vi "Event Handler.vi"(0 "uService Template in":refnum<class "Kasli Server.lvclass">, 5 "Event type":T1=enum."Message", 7 "Item Name":string, 9 "Data":variant, 11 "error in (no error)":errorcluster) -> (4 "uService Template out":refnum<class "Kasli Server.lvclass">, 15 "error out":errorcluster)   [LabVIEW 2020, in "Kasli Server.lvlib" / "Kasli Server.lvclass"]
uses:
  Kasli Server.lvclass
  C:/Users/marco/Documents/GitHub_Lab/TALOS/talos/Father of all uServices/Father of all uServices/Father of all uServices.lvclass
  Father of all uServices/Father of all uServices/Event Handler Items.ctl
  Ancestor/Ancestor/Ancestor.lvclass/Ancestor.ctl
  Kasli Server Consumer Case Selector.ctl
  Father of all uServices/Father of all uServices Messages/Consumer Msg/Consumer Msg.lvclass/Consumer Msg.ctl
  FGV/Error Memory/Get Error Description.vi
  Support VIs/Get PC name.vi
  Ancestor/Ancestor/Read ID.vi
  Support VIs/Get Class Name.vi
  <vilib>/Utility/error.llb/Clear Errors.vi
  Father of all uServices/Father of all uServices Messages/Consumer Msg/Send Consumer.vi
  Support VIs/Substitute Error.vi
  FGV/Error Memory/Error Memory Core.vi
  <vilib>/AdvancedString/Delimited String to 1D String Array.vi
  Support VIs/Circus Root Path.vi
  FGV/Error Memory/Error Crt Lvl checker.vi
  FGV/Error Memory/Error Memory Core.vi/40c8088d-b597-4017-91af-faa98e00292e.vi
  FGV/Error Memory/Error Memory Core.vi/d4a3ab98-063c-4e44-b43d-fbdcfe6c2be2.vi
  Father of all uServices/Father of all uServices/Father of all uServices.lvclass
  C:/Users/marco/Documents/GitHub_Lab/TALOS/builds/Actor Framework PPL/Actor Framework.lvlibp/1abvi3w/vi.lib/ActorFramework/Actor/Actor.lvclass
  Support VIs/Global Memory.vi
  <vilib>/Utility/LVClass/Get LV Class Name.vi
  Support VIs/Is in Packed Library.vi
  Support VIs/TALOS Root path.vi
  Support VIs/Read CSV worksheet.vi
  Support VIs/Global Constants.vi
  <vilib>/Utility/error.llb/General Error Handler.vi
  Father of all uServices/Father of all uServices/Children Methods/Get GUI Item Value - String.vi
  builds/Actor Framework PPL/Actor Framework.lvlibp/1abvi3w/vi.lib/ActorFramework/Actor/Read Self Enqueuer.vi
  <userlib>/_OpenG.lib/lvdata/lvdata.llb/Get Strings from Enum__ogtk.vi
  builds/Actor Framework PPL/Actor Framework.lvlibp/1abvi3w/vi.lib/ActorFramework/Message Enqueuer/Enqueue.vi
  Support VIs/Error Log.vi
  Ancestor/Ancestor/Ancestor.lvclass
  <vilib>/Comparison/Equal/Equal Functor/Equal Functor.lvclass
  Father of all uServices/Father of all uServices Messages/Consumer Msg/Consumer Msg.lvclass
  TALOS.lvlib
  C:/Users/marco/Documents/GitHub_Lab/TALOS/talos/Ancestor/Ancestor/Ancestor.lvclass
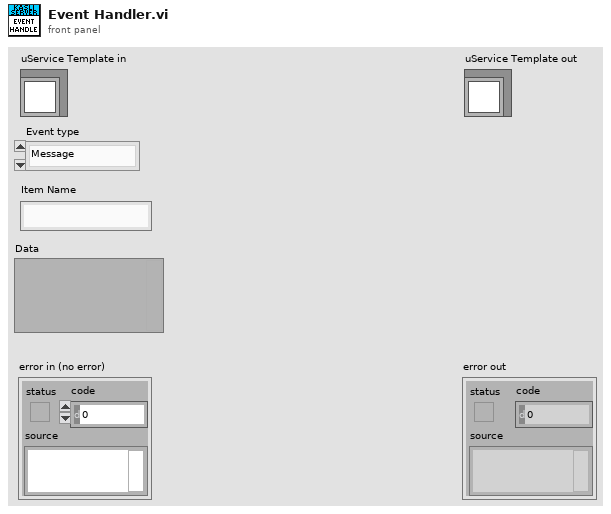
[diagram p1: front panel]
types:
  T1 = typedef "TALOS.lvlib/Father of all uServices.lvlib/Father of all uServices.lvclass/Event Handler Items.ctl" = enum16{"Button Pressed", "Shared Variable Updated", "Message", "Ready to launch?", "Safe Mode", "Start RUN", "Stop RUN"}
  T2 = typedef "Kasli Server.lvlib/Kasli Server.lvclass/Kasli Server Consumer Case Selector.ctl" = enum16{"Send Message to Kasli"}
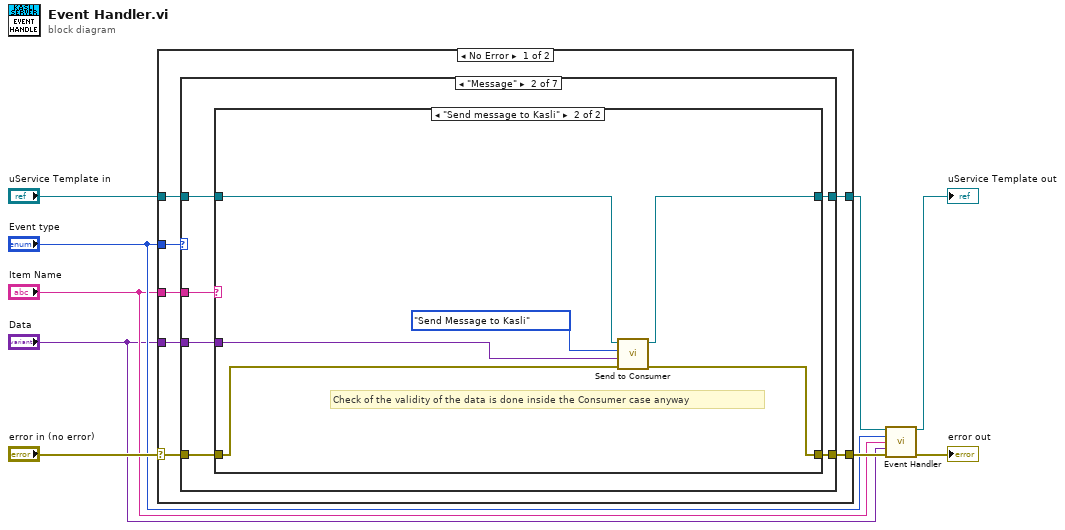
[diagram p0: block diagram]
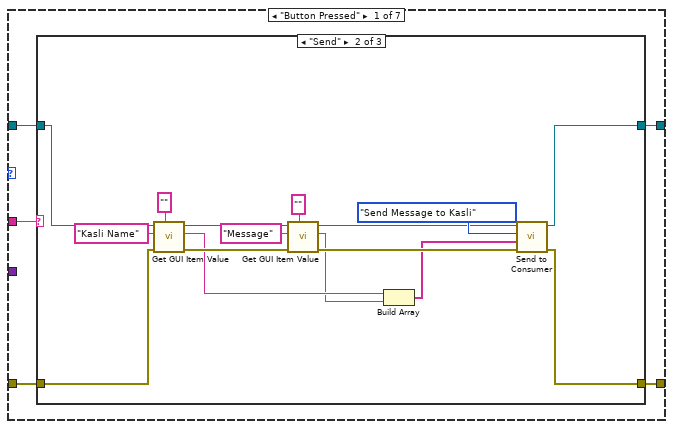
[diagram p2: hidden frame]
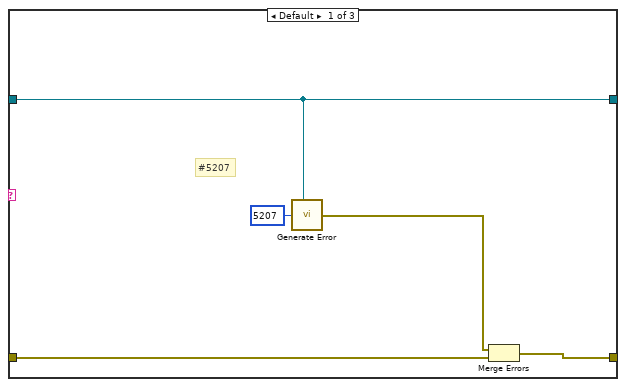
[diagram p3: hidden frame]
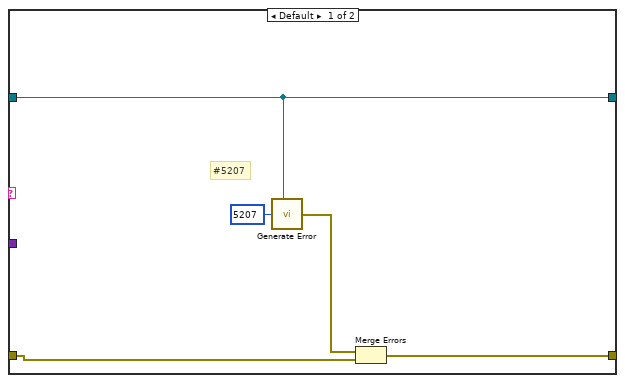
[diagram p5: hidden frame]
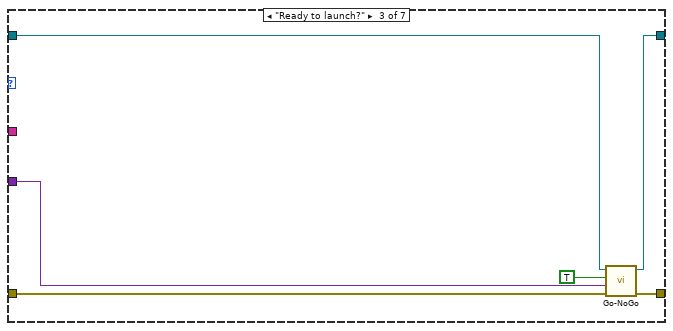
[diagram p6: hidden frame]
diagram:
  n1 = case shown="No Error" "error in (no error)" {
    selector: "error in (no error)" -> [w13 w77]
    tunnel: [w12 w77] -> w7
    tunnel: "uService Template in" -> [w15 w76]
    tunnel: [w14 w76] -> w4
    tunnel: "Event type" -> [w16 _]
    tunnel: "Item Name" -> [w11 _]
    tunnel: "Data" -> [w10 _]
    frame No Error {
      n2 = case shown="\"Message\"" w16 {
        tunnel: w15 -> [w21 w50 w64 w69 w71 w73 w75]
        tunnel: [w20 w46 w67 w69 w71 w73 w75] -> w14
        tunnel: w13 -> [w17 w47 w65 w68 w70 w72 w74]
        tunnel: [w18 w45 w66 w68 w70 w72 w74] -> w12
        tunnel: w11 -> [w19 w49 _ _ _ _ _]
        tunnel: w10 -> [_ w48 w62 _ _ _ _]
        frame "Button Pressed" {
          n3 = case shown="\"Send\"" w19 {
            tunnel: w21 -> [w22 w37 w44]
            tunnel: [w22 w34 w44] -> w20
            tunnel: [w25 w27 w43] -> w18
            tunnel: w17 -> [w26 w31 w43]
            frame Default {
              # "#5207"
              n4 = call "Generate Error.vi"("Class"=w22, "Error Code"=5207) -> ("error out"=w24:errorcluster)  [unwired: 5 in]
              n5 = Merge Errors(w24, w26) -> (w25:errorcluster)
            }
            frame "Send" {
              n6 = call-poly "Get GUI Item Value.vi"("Default"="", "error in (no error)"=w31, "FP Item Name"="Kasli Name", "uService Template in"=w37) -> ("error out"=w39:errorcluster, "Value"=w30:string, "uService Template out"=w36:refnum<class "Kasli Server.lvclass">)  [unwired: 5 in]
              n7 = call-poly "Get GUI Item Value.vi"("Default"="", "error in (no error)"=w39, "FP Item Name"="Message", "uService Template in"=w36) -> ("error out"=w38:errorcluster, "Value"=w29:string, "uService Template out"=w35:refnum<class "Kasli Server.lvclass">)  [unwired: 5 in]
              n8 = Build Array(w30, w29) -> (w28:string[])
              n9 = call "Send to Consumer.vi"("error in (no error)"=w38, "Data"=w28, "Case ID"=Kasli_Server_Consumer_Case_Selector."Send Message to Kasli" ("Kasli Server Consumer Case Selector"), "uService Template in"=w35) -> ("error out"=w27:errorcluster, "uService Template out"=w34:refnum<class "Kasli Server.lvclass">)  [unwired: 6 in]
            }
            frame "Example" {
            }
          }
        }
        frame "Message" {
          n10 = case shown="\"Send message to Kasli\"" w49 {
            tunnel: w50 -> [w53 w57]
            tunnel: w48 -> [_ w61]
            tunnel: w47 -> [w51 w60]
            tunnel: [w53 w58] -> w46
            tunnel: [w52 w59] -> w45
            frame Default {
              # "#5207"
              n11 = call "Generate Error.vi"("Class"=w53, "Error Code"=5207) -> ("error out"=w54:errorcluster)  [unwired: 5 in]
              n12 = Merge Errors(w54, w51) -> (w52:errorcluster)
            }
            frame "Send message to Kasli" {
              # "Check of the validity of the data is done inside the Consumer case anyway"
              n13 = call "Send to Consumer.vi"("error in (no error)"=w60, "Data"=w61, "Case ID"=Kasli_Server_Consumer_Case_Selector."Send Message to Kasli" ("Kasli Server Consumer Case Selector"), "uService Template in"=w57) -> ("error out"=w59:errorcluster, "uService Template out"=w58:refnum<class "Kasli Server.lvclass">)  [unwired: 6 in]
            }
          }
        }
        frame "Ready to launch?" {
          n14 = call-dynamic "Go-NoGo.vi"("error in (no error)"=w65, "Go-NoGo Data"=w62, "Go?"=TRUE, "Father of all uServices in"=w64) -> ("error out"=w66:errorcluster, "Father of all uServices out"=w67:refnum<class "Kasli Server.lvclass">)  [unwired: 6 in]
        }
        frame "Safe Mode" {
        }
        frame "Start RUN" {
        }
        frame "Stop RUN" {
        }
        frame "Shared Variable Updated" {
        }
      }
    }
    frame Error {
    }
  }
  n15 = call-parent "Event Handler.vi"("uService Template in"=w4, "Event type"="Event type", "Item Name"="Item Name", "Data"="Data", "error in (no error)"=w7) -> ("uService Template out"=→"uService Template out":refnum<class "Kasli Server.lvclass">, "error out"=→"error out":errorcluster)  [unwired: 9 in]
